vi "Make JSON Array.vi"(6 "Pretty Print?":bool, 8 "error in (no error)":errorcluster, 9 "Array of JSON Text":string[](array[string])) -> (0 "error out":errorcluster, 3 "<JSON>Array":string)   [LabVIEW 2015, in "JSONtext.lvlib"]
doc: "Format a JSON Array out of an array of JSON items."
uses:
  JSONtext.lvlib
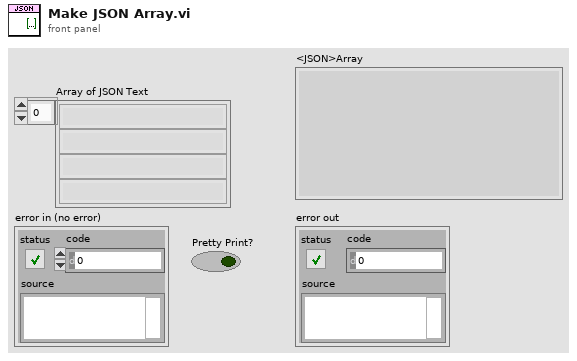
[diagram p1: front panel]
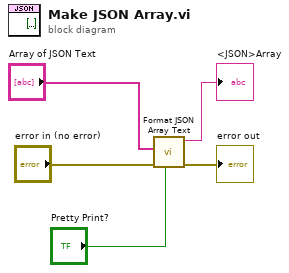
[diagram p0: block diagram]
diagram:
  n1 = call "Format JSON Array Text.vi"("Pretty Print?"="Pretty Print?", "error in (no error)"="error in (no error)", "Array of JSON Text"="Array of JSON Text") -> ("error out"=→"error out":errorcluster, "<JSON>"=→"<JSON>Array":string)  [unwired: 7 in]
